vi "GluePattern_olddraft(SubVI).vi"(5 "File to be processed- Dots":path=path "C:/Users/Aerotech/Documents/BNL_ThermomechanicalStave/1_ModulePlacement/1_GluePatterning/LabVIEW_gluepattern_arraytest.csv", 6 "Type of Pattern":u16(ring) items=["Dots", "Lines"], 7 "Go to \ncoordinates":T5={"X [mm]"=10.0, "Y [mm]"=-17.0, "Z [mm] "=36.0}) -> ()   [LabVIEW 2016]
uses:
  C:/Users/Aerotech/Documents/BNL_ThermomechanicalStave/AerotechLibraries/Bin/Aerotech.A3200.dll
  AerotechLibraries/Bin/Aerotech.A3200.dll
  <vilib>/LabVIEW Interface for Arduino/Type Defs/Arduino Resource.ctl
  <vilib>/LabVIEW Interface for Arduino/Type Defs/Board Type.ctl
  <vilib>/LabVIEW Interface for Arduino/Type Defs/Pin Mode.ctl
  <vilib>/Utility/file.llb/Read Delimited Spreadsheet (DBL).vi
  <vilib>/LabVIEW Interface for Arduino/LabVIEW Interface for Arduino.lvlib
panel:
  in  "Error In":errorcluster
  out "Arduino Resource":T1={"VISA resource"="COM3", "Board Type"=enum."Uno", "Connection Type"=enum."USB / Serial", "Bytes Per Packet (15)"=15}
  in  "Digital I/O Pin":u8=7
  out "error out":errorcluster
  out "DX [mm]":dbl
  out "DY [mm]":dbl
  in  "Final Z":dbl=41.0
  out "Final Position":T3={"Final X"=10.000061631047261, "Final Y"=-16.999877872052817, "Final Z"=35.999801000000005}
  out "Column":i32
  out "Row":i32
  in  "Home?":bool
  out "XYZ Stage Control":refnum<k24>
  in  "Axis Speeds":T4={"vX [mm]"=40.0, "vY [mm]"=40.0, "vZ [mm] "=40.0}
  in  "Module width [mm]":dbl
  in  "Module length [mm]":dbl
  out "INPUT : Dot":bool[][](array[boolean])=[[TRUE]]
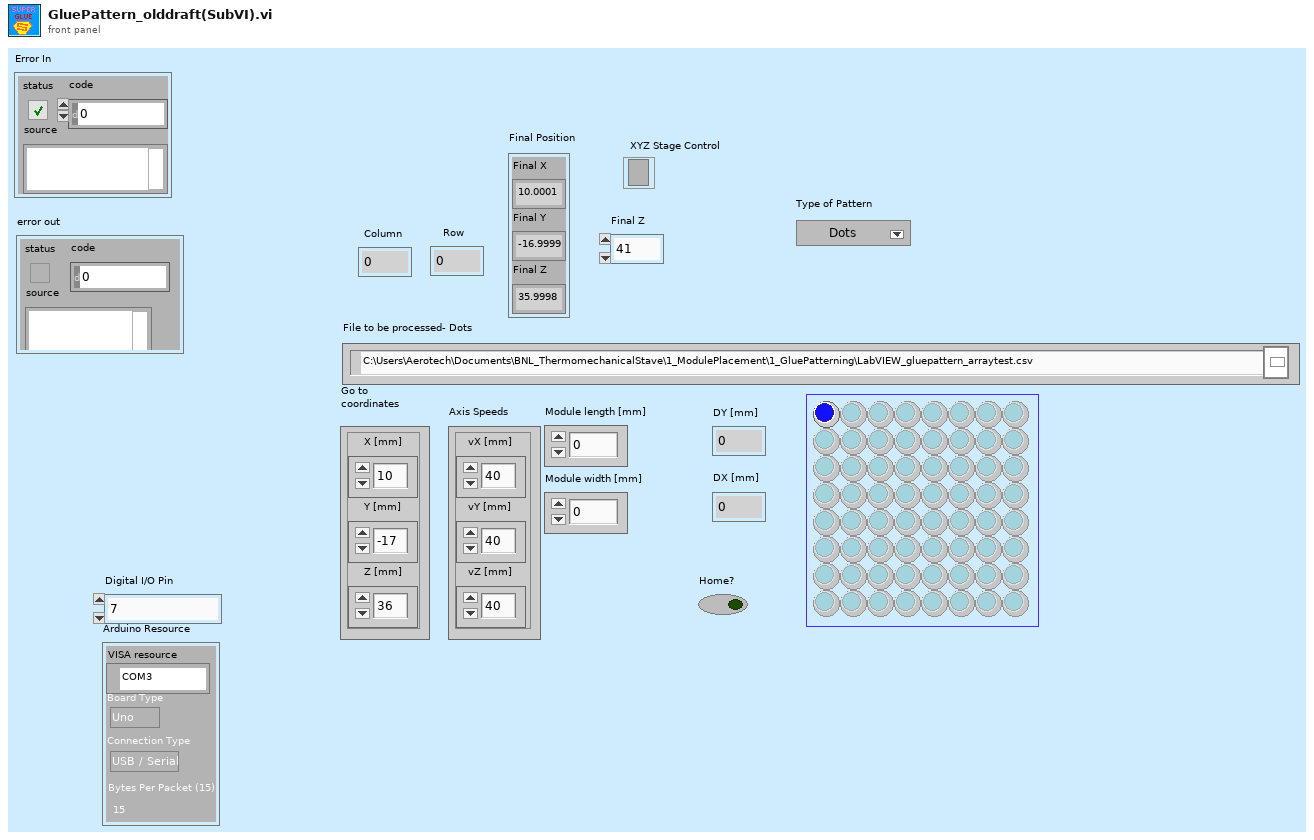
[diagram p1: front panel]
types:
  T1 = typedef "LabVIEW Interface for Arduino.lvlib/Arduino Resource.ctl" = cluster{"VISA resource":refnum<visa-resource-name>, "Board Type":T2, "Connection Type":enum8{"USB / Serial"}, "Bytes Per Packet (15)":u8}
  T2 = typedef "LabVIEW Interface for Arduino.lvlib/Board Type.ctl" = enum16{"Uno", "Dimuelanove w/Atmega 328", "Mega 2560"}
  T3 = cluster{"Final X":dbl, "Final Y":dbl, "Final Z":dbl}
  T4 = cluster{"vX [mm]":dbl, "vY [mm]":dbl, "vZ [mm] ":dbl}
  T5 = cluster{"X [mm]":dbl, "Y [mm]":dbl, "Z [mm] ":dbl}
  T6 = typedef "LabVIEW Interface for Arduino.lvlib/Pin Mode.ctl" = enum8{"Input", "Output"}
  T7 = cluster{"X [mm]":dbl, "Y [mm]":dbl, "Z [mm]":dbl}
  T8 = cluster{"X Position Feedback":dbl, "Y Position Feedback":dbl, "Z Position Feedback":dbl}
  T9 = cluster{"Final X":dbl, "Final Y":dbl, "Z [mm] ":dbl}
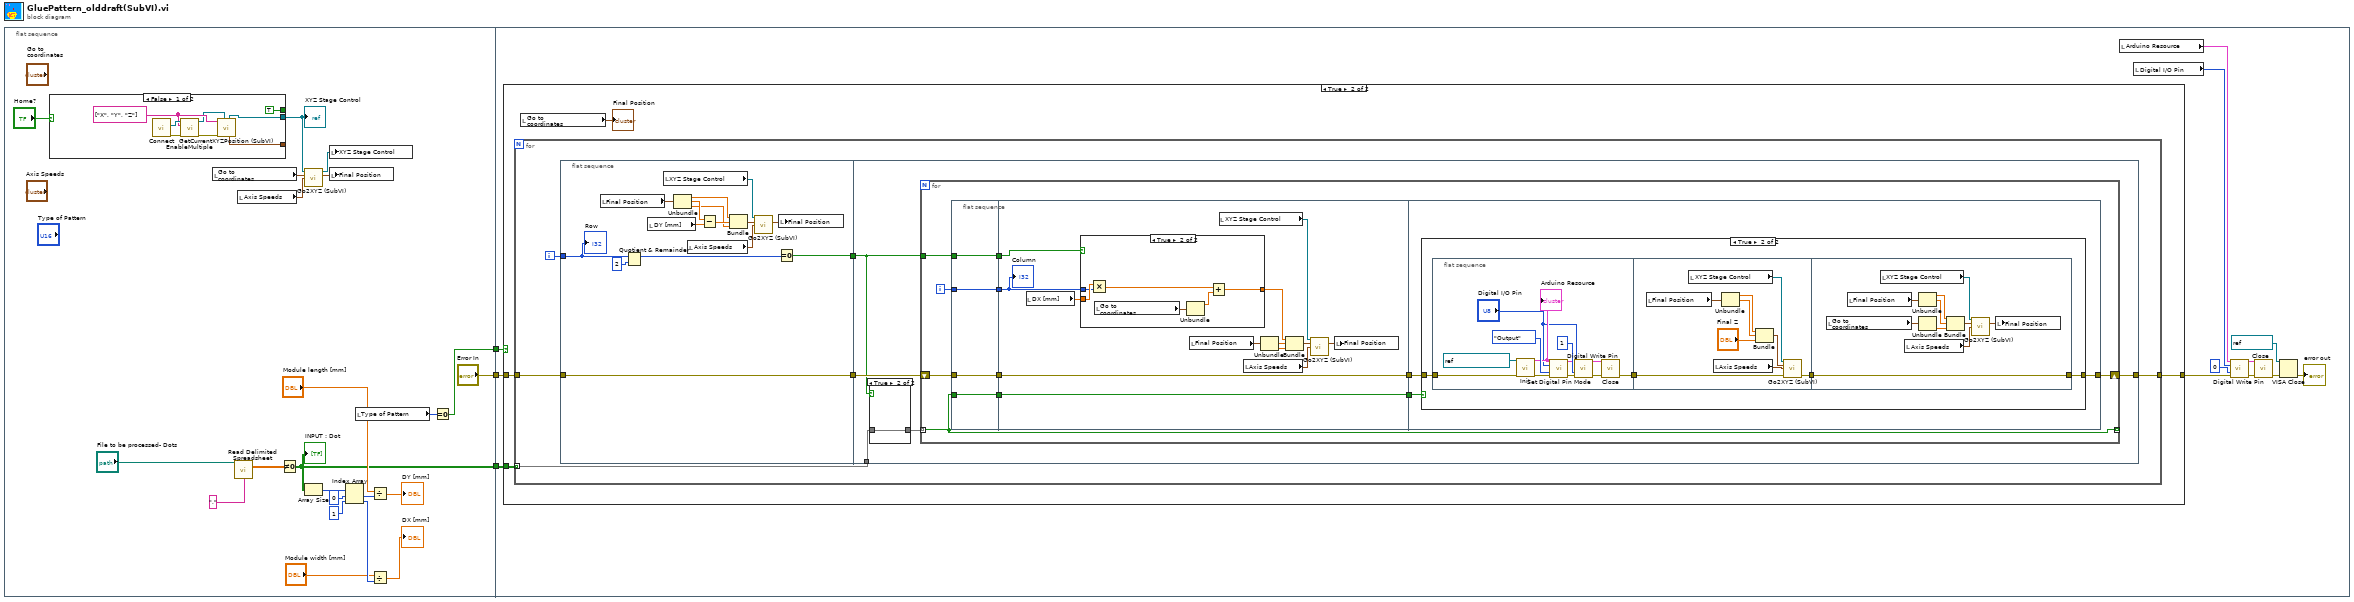
[diagram p0: block diagram]
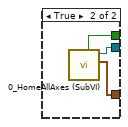
[diagram p2: hidden frame]
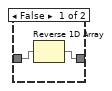
[diagram p4: hidden frame]
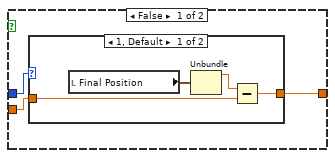
[diagram p5: hidden frame]
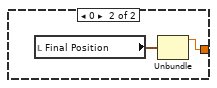
[diagram p6: hidden frame]
diagram:
  n1 = flat-sequence {
    tunnel: ["Error In"] -> w3
    tunnel: [w5] -> w2
    tunnel: [w6] -> w1
    tunnel: w3 -> [w48]
    tunnel: w2 -> [w47]
    tunnel: w1 -> [w46]
    frame #0 {
      n2 = case shown="False" "Home?" {
        tunnel: [w26 w36] -> _
        tunnel: [TRUE ("completed") w35] -> _
        tunnel: [w28 w34] -> w13
        frame False {
          w30 = string[] ["X", "Y", "Z"] ("Axes Names")
          n3 = call "Connect.vi"() -> ("error out"=w32:errorcluster, "controller"=w31:refnum<k24>)  [unwired: 10 in]
          n4 = call "EnableMultiple.vi"("error in (no error)"=w32, "axis names"=w30, "controller in"=w31) -> ("error out"=w33:errorcluster, "controller out"=w29:refnum<k24>)  [unwired: 7 in]
          n5 = call "GetCurrentXYZPosition (SubVI).vi"(".NET Refnum in - Device"=w29, "error in (no error)"=w33, "Axes Names"=w30) -> ("Current stage position"=w26:T7, ".NET Refnum out  - Device"=w28:refnum<k24>)  [unwired: 3 in, 4 out]
        }
        frame True {
          n6 = call "0_HomeAllAxes (SubVI).vi"() -> ("Homed coordinates"=w36:T8, "controller out"=w34:refnum<k24>, "completed"=w35:bool)  [unwired: 8 in, 1 out]
        }
      }
      "XYZ Stage Control" <- w13
      n7 = local read "Go to \ncoordinates"() -> (w8:T5)
      n8 = call-poly <vilib>:"Read Delimited Spreadsheet.vi"("file path (dialog if empty)"="File to be processed- Dots", "delimiter (\\t)"="," ("delimiter (\\t)")) -> ("all rows"=w24:dbl[][])  [unwired: 8 in, 5 out]
      n9 = local read "Axis Speeds"() -> (w10:T4)
      n10 = Not Equal To 0?(x=w24) -> (x != 0?=w5:bool[][])
      "INPUT : Dot" <- w5
      n11 = call "Go2XYZ (SubVI).vi"(".NET Refnum in"=w13, "Go to Coordinates"=w8, "Axis Speeds"=w10) -> (".NET Refnum out"=w9:refnum<k24>, "Final Position"=w11:T3)  [unwired: 8 in, 3 out]
      n12 = Array Size(array=w5) -> (size(s)=w23:i32[])
      n13 = local write "XYZ Stage Control"(w9) -> ()
      n14 = local write "Final Position"(w11) -> ()
      n15 = Index Array(array=w23, index #1=0 ("index"), index #2=1 ("index")) -> (element #1=w19:i32, element #2=w18:i32)
      n16 = local read "Type of Pattern"() -> (w7:u16)
      n17 = Divide(x="Module length [mm]", y=w19) -> (x/y=→"DY [mm]":dbl)
      n18 = Divide(x="Module width [mm]", y=w18) -> (x/y=→"DX [mm]":dbl)
      n19 = Equal To 0?(x=w7) -> (x = 0?=w6:bool)
    }
    frame #1 {
      n20 = case shown="True" w46 {
        tunnel: w47 -> [_ w53]
        tunnel: [w49 w52] -> w41
        tunnel: w48 -> [w49 w51]
        frame False {
        }
        frame True {
          n21 = for {
            tunnel: w53 -> [w54] mode=indexing
            tunnel: [w58] -> w52
            tunnel: w51 -> [w56]
            i -> [w59]
            n22 = flat-sequence {
              tunnel: w59 -> [w63]
              tunnel: [w74] -> w57
              tunnel: w56 -> [w74]
              tunnel: [w60] -> w55
              tunnel: w54 -> [w77]
              tunnel: [w79] -> w58
              tunnel: w57 -> [w78]
              tunnel: w55 -> [w75]
              frame #0 {
                n23 = local read "Final Position"() -> (w68:T3)
                n24 = Quotient & Remainder(x=w63, y=2) -> (x-y*floor(x/y)=w61:i32)  [unwired: 1 out]
                n25 = local read "DY [mm]"() -> (w64:dbl)
                n26 = local read "XYZ Stage Control"() -> (w66:refnum<k24>)
                n27 = Unbundle(w68) -> ("Final X"=w69:dbl, "Final Y"=w71:dbl, "Final Z"=w70:dbl)
                n28 = local read "Axis Speeds"() -> (w73:T4)
                n29 = Subtract(x=w71, y=w64) -> (x-y=w72:dbl)
                n30 = Bundle("Final X"=w69, w72, "Final Z"=w70) -> (w67:cluster{"Final X":dbl, dbl, "Final Z":dbl})  [unwired: 1 in]
                n31 = call "Go2XYZ (SubVI).vi"(".NET Refnum in"=w66, "Go to Coordinates"=w67, "Axis Speeds"=w73) -> ("Final Position"=w65:T3)  [unwired: 8 in, 4 out]
                n32 = Equal To 0?(x=w61) -> (x = 0?=w60:bool)
                n33 = local write "Final Position"(w65) -> ()
                "Row" <- w63
              }
              frame #1 {
                n34 = case shown="True" w75 {
                  tunnel: w77 -> [w81 w82]
                  tunnel: [w80 w82] -> w76
                  frame False {
                    n35 = Reverse 1D Array(array=w81) -> (reversed array=w80:bool[])
                  }
                  frame True {
                  }
                }
                n36 = for {
                  shift-right: [w89] -> w79
                  shift-left: w78 -> [w92]
                  tunnel: [w83] -> _ mode=indexing
                  tunnel: w75 -> [w88]
                  tunnel: w76 -> [w83] mode=indexing
                  i -> [w93]
                  n37 = flat-sequence {
                    tunnel: w88 -> [w94]
                    tunnel: w83 -> [w95]
                    tunnel: w92 -> [w96]
                    tunnel: w93 -> [w97]
                    tunnel: [w97] -> w87
                    tunnel: [w96] -> w86
                    tunnel: [w95] -> w85
                    tunnel: [w94] -> w84
                    tunnel: [w106] -> w91
                    tunnel: [w98] -> w90
                    tunnel: w87 -> [w107]
                    tunnel: w86 -> [w106]
                    tunnel: w85 -> [w98]
                    tunnel: w84 -> [w99]
                    tunnel: w91 -> [w128]
                    tunnel: w90 -> [w126]
                    tunnel: [w127] -> w89
                    frame #0 {
                    }
                    frame #1 {
                      n38 = local read "DX [mm]"() -> (w108:dbl)
                      n39 = case shown="True" w99 {
                        tunnel: w108 -> [w112 w125]
                        tunnel: w107 -> [w111 w120]
                        tunnel: [w113 w121] -> w100
                        frame False {
                          n40 = case shown="1, Default" w111 {
                            tunnel: [w117 w118] -> w113
                            tunnel: w112 -> [w116 _]
                            frame 1, Default {
                              n41 = local read "Final Position"() -> (w115:T3)
                              n42 = Unbundle(w115) -> ("Final X"=w114:dbl)  [unwired: 2 out]
                              n43 = Subtract(x=w114, y=w116) -> (x-y=w117:dbl)
                            }
                            frame 0 {
                              n44 = local read "Final Position"() -> (w119:T3)
                              n45 = Unbundle(w119) -> ("Final X"=w118:dbl)  [unwired: 2 out]
                            }
                          }
                        }
                        frame True {
                          n46 = Multiply(x=w125, y=w120) -> (x*y=w123:dbl)
                          n47 = local read "Go to \ncoordinates"() -> (w124:T5)
                          n48 = Unbundle(w124) -> ("X [mm]"=w122:dbl)  [unwired: 2 out]
                          n49 = Add(x=w123, y=w122) -> (x+y=w121:dbl)
                        }
                      }
                      n50 = local read "Final Position"() -> (w105:T3)
                      n51 = local read "XYZ Stage Control"() -> (w109:refnum<k24>)
                      n52 = local read "Axis Speeds"() -> (w110:T4)
                      n53 = Unbundle(w105) -> ("Final Y"=w104:dbl, "Final Z"=w101:dbl)  [unwired: 1 out]
                      n54 = Bundle("Final X"=w100, "Final Y"=w104, "Final Z"=w101) -> (w102:T3)  [unwired: 1 in]
                      n55 = call "Go2XYZ (SubVI).vi"(".NET Refnum in"=w109, "Go to Coordinates"=w102, "Axis Speeds"=w110) -> ("Final Position"=w103:T3)  [unwired: 8 in, 4 out]
                      n56 = local write "Final Position"(w103) -> ()
                      "Column" <- w107
                    }
                    frame #2 {
                      n57 = case shown="True" w126 {
                        tunnel: [w129 w132] -> w127
                        tunnel: w128 -> [w129 w133]
                        frame False {
                        }
                        frame True {
                          n58 = flat-sequence {
                            tunnel: w133 -> [w135]
                            tunnel: [w142] -> w130
                            tunnel: [w146] -> w131
                            tunnel: w130 -> [w147]
                            tunnel: [w155] -> w132
                            tunnel: w131 -> [w155]
                            frame #0 {
                              n59 = call <vilib>:"Init.vi"("VISA resource"=refnum<visa-resource-name> "COM3", "error in"=w135) -> ("Arduino Resource"=w138:T1, "error out"=w139:errorcluster)  [unwired: 16 in]
                              "Arduino Resource" <- w138
                              n60 = call <vilib>:"Set Digital Pin Mode.vi"("Arduino Resource"=w138, "Digital I/O Pin"="Digital I/O Pin", "Pin Mode (Input)"=Pin_Mode."Output", "error in"=w139) -> ("Arduino Resource"=w137:T1, "error out"=w136:errorcluster)  [unwired: 10 in]
                              n61 = call <vilib>:"Digital Write Pin.vi"("Arduino Resource"=w137, "Digital I/O Pin (0)"="Digital I/O Pin", "Value (0)"=u8 1, "error in"=w136) -> ("Arduino Resource"=w144:T1, "error out"=w143:errorcluster)  [unwired: 10 in]
                              n62 = call <vilib>:"Close.vi"("Arduino Resource"=w144, "error in"=w143) -> ("error out"=w142:errorcluster)  [unwired: 13 in]
                            }
                            frame #1 {
                              n63 = local read "Final Position"() -> (w150:T3)
                              n64 = local read "XYZ Stage Control"() -> (w152:refnum<k24>)
                              n65 = local read "Axis Speeds"() -> (w153:T4)
                              n66 = Unbundle(w150) -> ("Final X"=w149:dbl, "Final Y"=w148:dbl)  [unwired: 1 out]
                              n67 = Bundle("Final X"=w149, "Final Y"=w148, "Final Z"="Final Z") -> (w151:T3)  [unwired: 1 in]
                              n68 = call "Go2XYZ (SubVI).vi"(".NET Refnum in"=w152, "Go to Coordinates"=w151, "Axis Speeds"=w153, "error in (no error)"=w147) -> ("error out"=w146:errorcluster)  [unwired: 7 in, 4 out]
                            }
                            frame #2 {
                              n69 = local read "Go to \ncoordinates"() -> (w163:T5)
                              n70 = local read "Final Position"() -> (w164:T3)
                              n71 = local read "XYZ Stage Control"() -> (w157:refnum<k24>)
                              n72 = local read "Axis Speeds"() -> (w158:T4)
                              n73 = Unbundle(w164) -> ("Final X"=w162:dbl, "Final Y"=w161:dbl)  [unwired: 1 out]
                              n74 = Unbundle(w163) -> ("Z [mm]"=w160:dbl)  [unwired: 2 out]
                              n75 = Bundle("Final X"=w162, "Final Y"=w161, "Z [mm]"=w160) -> (w159:T9)  [unwired: 1 in]
                              n76 = call "Go2XYZ (SubVI).vi"(".NET Refnum in"=w157, "Go to Coordinates"=w159, "Axis Speeds"=w158) -> ("Final Position"=w156:T3)  [unwired: 8 in, 4 out]
                              n77 = local write "Final Position"(w156) -> ()
                            }
                          }
                        }
                      }
                    }
                  }
                }
              }
            }
          }
          n78 = local read "Go to \ncoordinates"() -> (→"Final Position":T5)
        }
      }
      n79 = local read "Arduino Resource"() -> (w38:T1)
      n80 = local read "Digital I/O Pin"() -> (w37:u8)
      n81 = call <vilib>:"Digital Write Pin.vi"("Arduino Resource"=w38, "Digital I/O Pin (0)"=w37, "Value (0)"=u8 0, "error in"=w41) -> ("Arduino Resource"=w43:T1, "error out"=w42:errorcluster)  [unwired: 10 in]
      n82 = call <vilib>:"Close.vi"("Arduino Resource"=w43, "error in"=w42) -> ("error out"=w40:errorcluster)  [unwired: 13 in]
      n83 = VISA Close(VISA resource name=refnum<visa-resource-name> "COM3", error in (no error)=w40) -> (error out=→"error out":errorcluster)
    }
  }
